vi "getZThXThYbow.vi"(8 "error in (no error)":errorcluster, 11 "PositionMeas in":refnum<class "PositionMeas.lvclass">) -> (0 "error out":errorcluster, 2 "Z,ThX,ThY,Bow_out":fxp<+/-,27,5>[](array[numeric]), 3 "PositionMeas out":refnum<class "PositionMeas.lvclass">)   [LabVIEW 2020, in "PositionMeas.lvclass"]
doc: "Returns the Z, ThX, ThY, and Bow measurements based on position sensor data"
uses:
  PositionMeas.lvclass
  PositionMeas.lvclass/PositionMeas.ctl
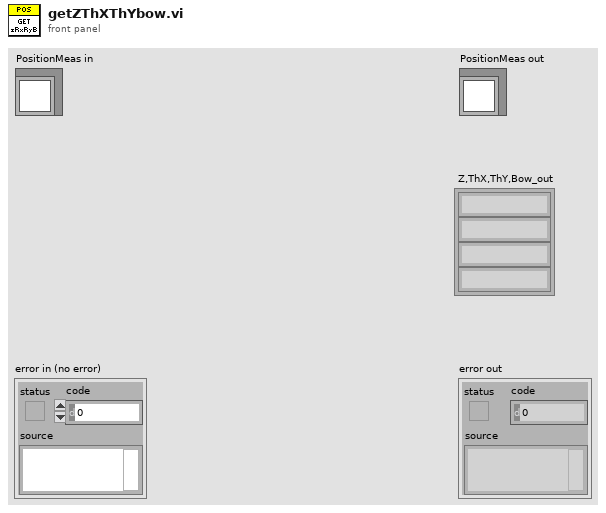
[diagram p1: front panel]
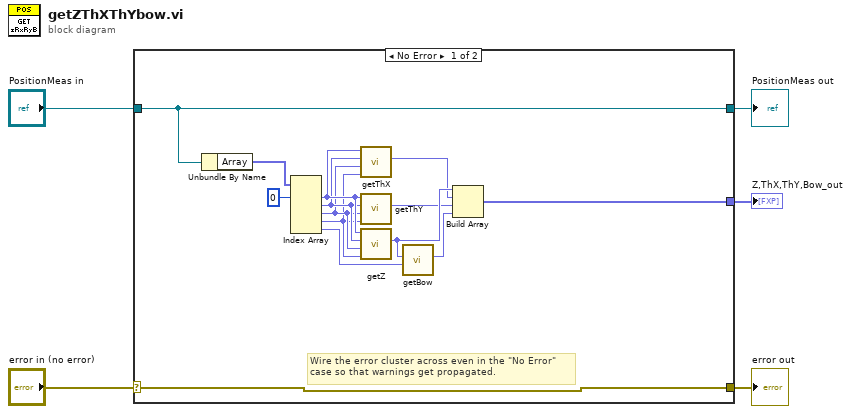
[diagram p0: block diagram]
diagram:
  n1 = case shown="No Error" "error in (no error)" {
    selector: "error in (no error)" -> [w19 w21]
    tunnel: [w19 w21] -> w4
    tunnel: [w18 w20] -> w2
    tunnel: "PositionMeas in" -> [w18 w20]
    tunnel: [w10 _] -> w1
    frame No Error {
      # "Wire the error cluster across even in the \"No Error\"\ncase so that warnings get propagated."
      n2 = Unbundle By Name(w18) -> ("Array"=w16:fxp<+/-,25,5>[])
      n3 = Index Array(array=w16, index #1=0 ("index")) -> (element #1=w15:fxp<+/-,25,5>, element #2=w14:fxp<+/-,25,5>, element #3=w13:fxp<+/-,25,5>, element #4=w12:fxp<+/-,25,5>, element #5=w11:fxp<+/-,25,5>)  [unwired: 4 in]
      n4 = call "getThX.vi"("SW"=w12, "NW"=w13, "NE"=w14, "SE"=w15) -> ("ThX"=w8:fxp<+/-,27,5>)  [unwired: 7 in]
      n5 = call "getThY.vi"("SW"=w12, "NW"=w13, "NE"=w14, "SE"=w15) -> ("ThY"=w7:fxp<+/-,27,5>)  [unwired: 7 in]
      n6 = call "getZ.vi"("SW"=w12, "NW"=w13, "NE"=w14, "SE"=w15) -> ("Z"=w9:fxp<+/-,27,5>)  [unwired: 7 in]
      n7 = call "getBow.vi"("CI"=w11, "Z"=w9) -> ("Bow"=w6:fxp<+/-,27,5>)  [unwired: 9 in]
      n8 = Build Array(w9, w8, w7, w6) -> (w10:fxp<+/-,27,5>[])
    }
    frame Error {
    }
  }
  "error out" <- w4
  "PositionMeas out" <- w2
  "Z,ThX,ThY,Bow_out" <- w1
